vi "subPrepConstellationPlots.vi"(10 "Oversample Factor":i32=16, 11 "Y":cdb[](array[numeric])) -> (3 "constellation graph":T1(array[cluster]) {"oversampled data" format="%.2f"; "constellation" format="%.2f"})   [LabVIEW 2011]
uses:
  <vilib>/addons/Modulation/Analog/controls/Complex Data Waveform.ctl
  <vilib>/addons/Modulation/niDMT.lvlib
  <vilib>/addons/Modulation/niAMT.lvlib
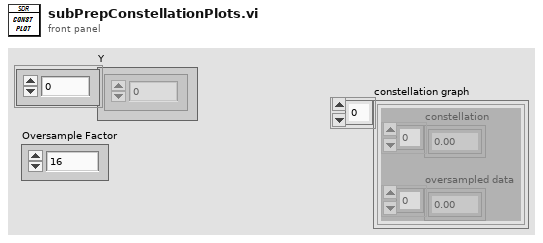
[diagram p1: front panel]
types:
  T1 = cluster{"constellation":dbl[], "oversampled data":dbl[]}[]
  T2 = typedef "niAMT.lvlib/Complex Data Waveform.ctl" = cluster{"t0":dbl, "dt":dbl, "Y":cdb[]}
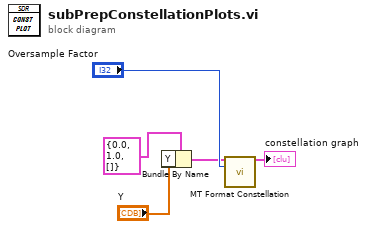
[diagram p0: block diagram]
diagram:
  n1 = Bundle By Name(cluster=T2 {"t0"=0.0, "dt"=1.0, "Y"=[]} ("waveform"), "Y"="Y") -> (w3:T2)
  n2 = call <vilib>:"MT Format Constellation.vi"("waveform"=w3, "samples per symbol"="Oversample Factor") -> ("constellation graph"=→"constellation graph":T1)  [unwired: 3 in, 10 out]
